vi "Read Name.vi"(8 "error in (no error)":errorcluster, 11 "Process In":refnum<class "Debug View.lvclass">) -> (0 "error out":errorcluster, 2 "Name":string, 3 "Process Out":refnum<class "Debug View.lvclass">)   [LabVIEW 2020, in "Debug View.lvclass"]
doc: "Returns the name of the object. The Qualified Name is prepended with the name of the owner recursively in the format \"Owner Name::Name\"."
uses:
  Debug View.lvclass
  Debug View.lvclass/Debug View.ctl
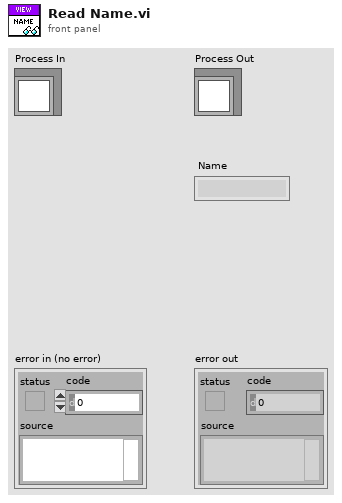
[diagram p1: front panel]
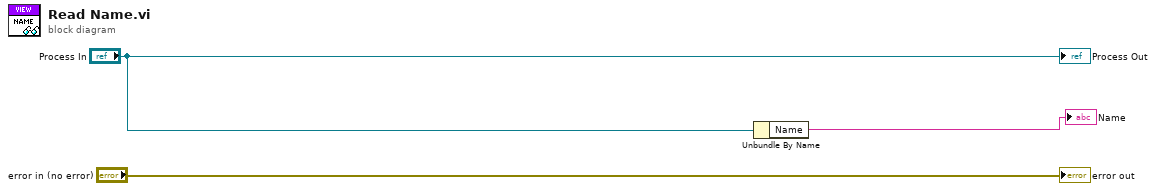
[diagram p0: block diagram]
diagram:
  n1 = Unbundle By Name("Process In") -> ("Name"=→"Name":string)
  "error out" <- "error in (no error)"
  "Process Out" <- "Process In"
